vi "NML Power Monitoring Main.vi"(0 "Initialize":bool, 1 "Start":bool, 2 "Data Directory":path=path "C:/Test/NML_PM_Monitoring/Data", 3 "UUT Serial Number(s)":string="12345", 5 "UUT COUNT":i32(ring) items=["1", "2", "3", "4", "5", "6"], 7 "HRS":dbl, 9 "MINS":dbl=5.0, 11 "INTERVAL":dbl=30.0 caption="PROFILER (SEC)", 12 "Stop":bool, 13 "PM 2936R Settings":T3={"Wavelength nm"=633, "Range Select"=1, "Mode"=0, "Unit Select"=2, "Auto Select"=1, "Analog Filter"=4, "Digital Filter\n(int. 0 to 10000)"=0, "Filter"=1} {"Filter" items=["No filtering", "Analog filter", "Digital filter", "Analog and Digital filter"]; "Digital Filter\n(int. 0 to 10000)" min=0 max=10000; "Analog Filter" items=["None", "250 kHz", "12.5 kHz", "1 kHz", "5 kHz"]; "Auto Select" items=["Manual Range", "Auto Range"]; "Unit Select" items=["Amps", "Volts", "Watts", "Watts/cm2", "Joules", "Joules/cm2", "dBm"]; "Mode" items=["CW Cont.", "DC Single", "Integrate", "Peak-to-Peak Cont.", "Peak-to-Peak Single", "Pulse Continuous", "Pulse Single", "RMS"]; "Range Select" items=["Range 0", "Range 1", "Range 2", "Range 3", "Range 4", "Range 5", "Range 6", "Range 7"]; "Wavelength nm" min=0}) -> (4 "Status Message":string, 6 "XY Plot - 1 Trace":cluster{"Seconds":dbl[], "Data Array":dbl[]}[](graph), 8 "# of Samples":i32=10, 10 "Acquired Samples":i32, 14 "Data":dbl[][](array[numeric]), 15 "Error Out":errorcluster)   [LabVIEW 2017]
uses:
  Commands.ctl
  C:/Program Files (x86)/Newport/Newport USB Driver/Bin/UsbDllWrap.dll
  Program Files (x86)/Newport/Newport USB Driver/Bin/UsbDllWrap.dll
  Newport PowerMeter 2936R/Device State Control.ctl
panel:
  out "Time Array":string[](array[string])
  out "Date Array":string[](array[string])
  out "Collecting\n    Data":bool
  out "Start Time":timestamp
  out "PM Ready":bool
  out "PM Count":i32
  out "MINS Left":dbl format="%_3g"
  out "HRS Left":dbl
  out "Data Graphs":T1(tab)
  out "XY Plot - 2 Traces":cluster{"Seconds":dbl[], "Data Array":dbl[]}[](graph)
  out "XY Plot - 3 Traces":cluster{"Seconds":dbl[], "Data Array":dbl[]}[](graph)
  out "XY Plot - 4 Traces":cluster{"Seconds":dbl[], "Data Array":dbl[]}[](graph)
  out "XY Plot - 5 Traces":cluster{"Seconds":dbl[], "Data Array":dbl[]}[](graph)
  out "XY Plot - 6 Traces":cluster{"Seconds":dbl[], "Data Array":dbl[]}[](graph)
  out "Sample":dbl[](array[numeric])
  in  "Error In":errorcluster
  out "PM Ref":refnum<k24>[](array[refnum])
  in  "Commands":T2
  # "RUN  TIME"
  # "INTERVALS"
  # "PROFILER (SEC)"
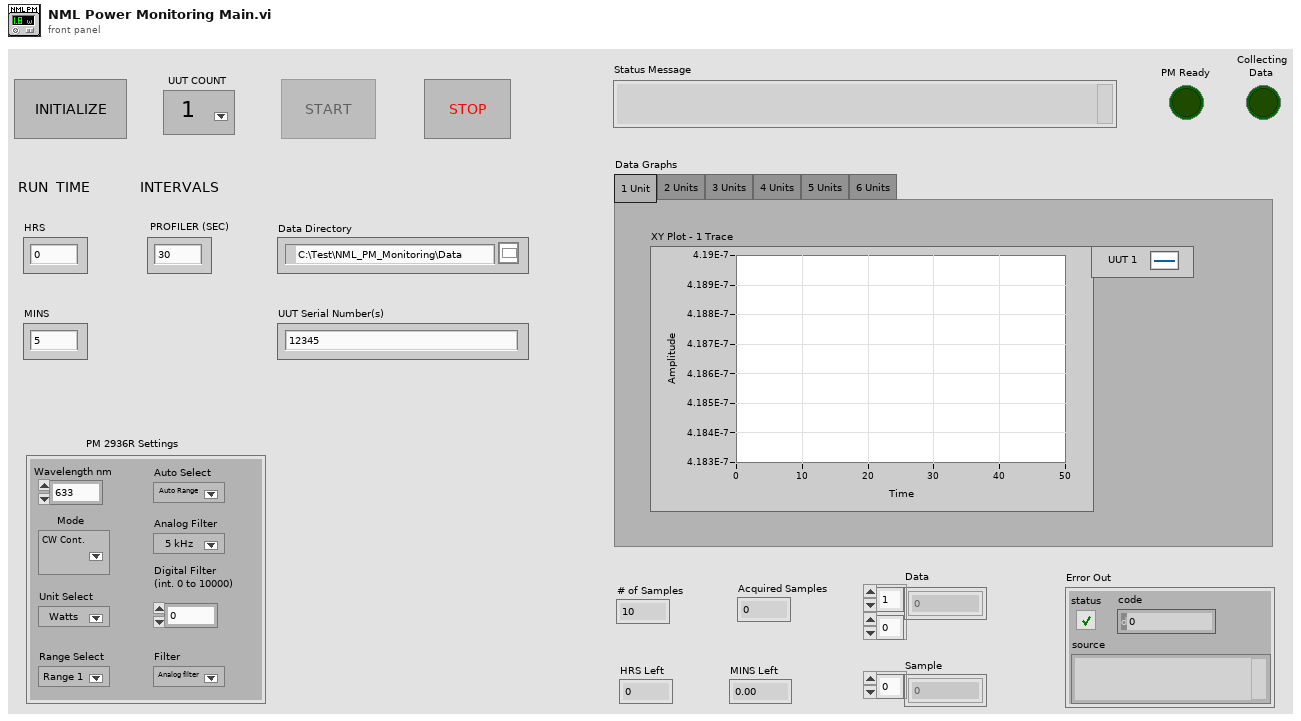
[diagram p1: front panel]
types:
  T1 = enum32{"1 Unit", "2 Units", "3 Units", "4 Units", "5 Units", "6 Units"}
  T2 = typedef "Commands.ctl" = enum16{"Idle", "Initialize", "Start", "Acquire Data", "Graph Data", "Store Data", "Halt"}
  T3 = cluster{"Wavelength nm":i32, "Range Select":i32, "Mode":i32, "Unit Select":i32, "Auto Select":i32, "Analog Filter":i32, "Digital Filter\n(int. 0 to 10000)":i32, "Filter":i32}
  T4 = enum8{"Enabled", "Disabled", "Disabled and Grayed Out"}
  T5 = typedef "Device State Control.ctl" = enum16{"Open", "Close", "Clear", "Set", "Reset", "Read", "Write", "Call"}
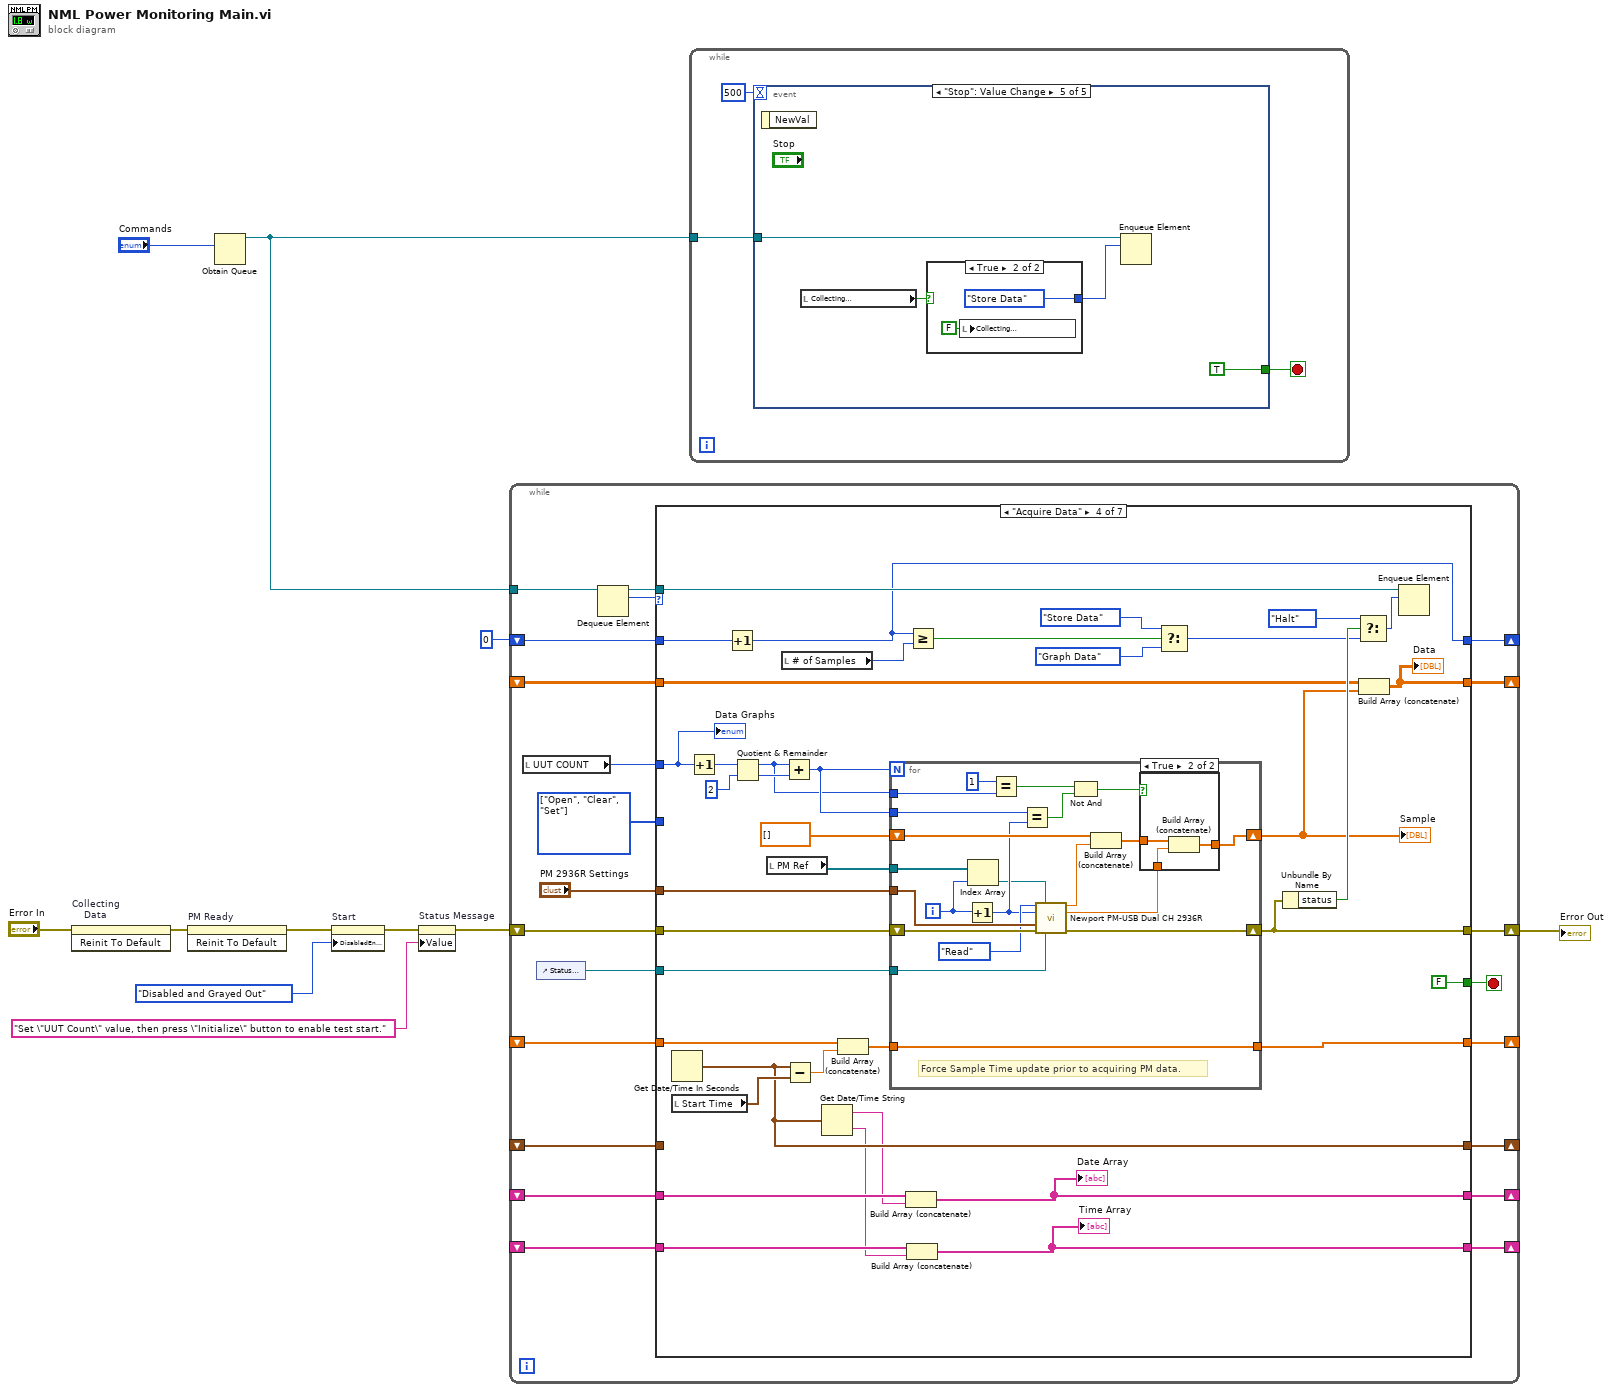
[diagram p0: block diagram]
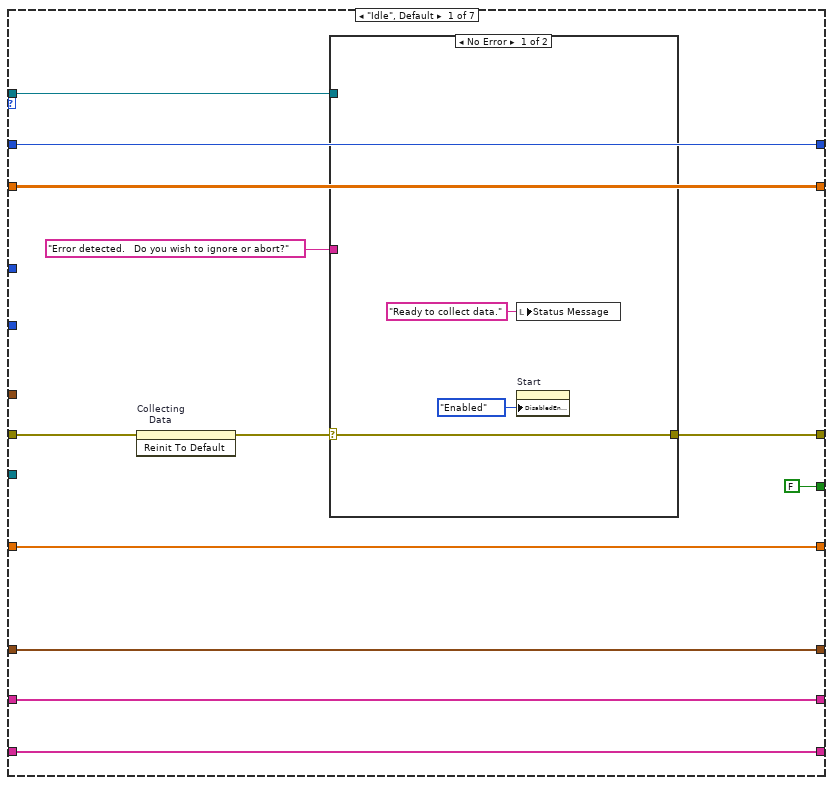
[diagram p2: hidden frame]
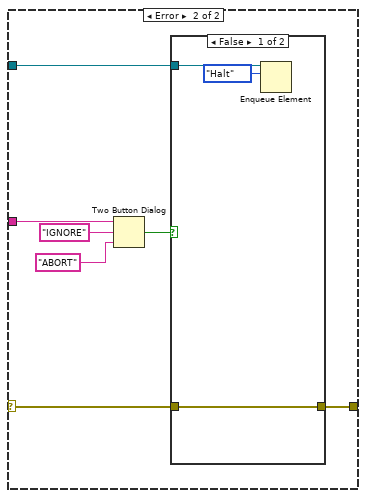
[diagram p3: hidden frame]
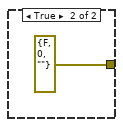
[diagram p4: hidden frame]
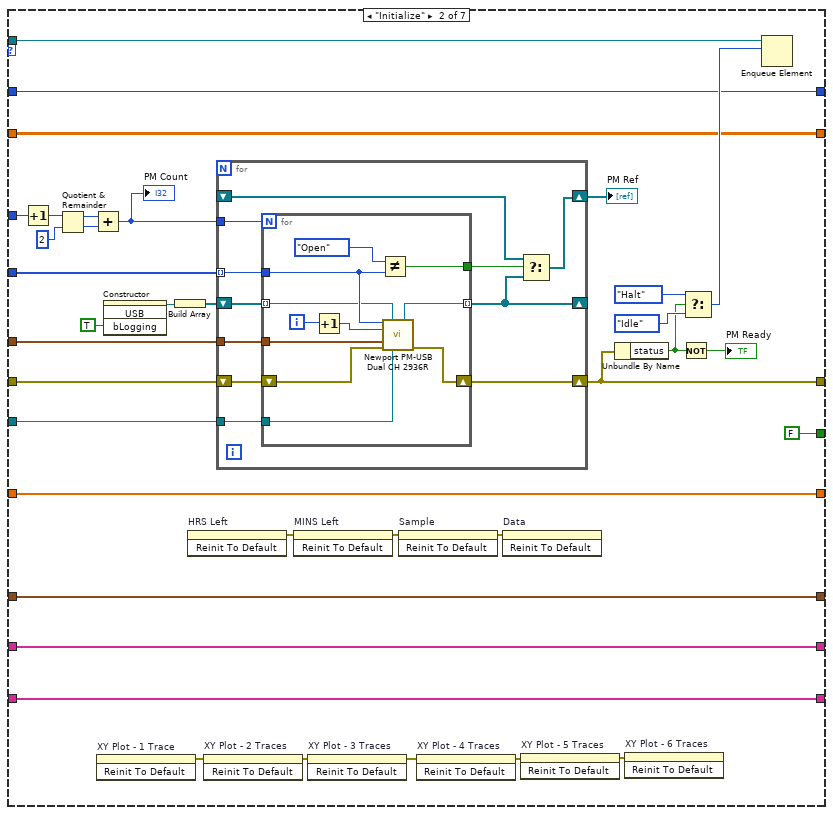
[diagram p5: hidden frame]
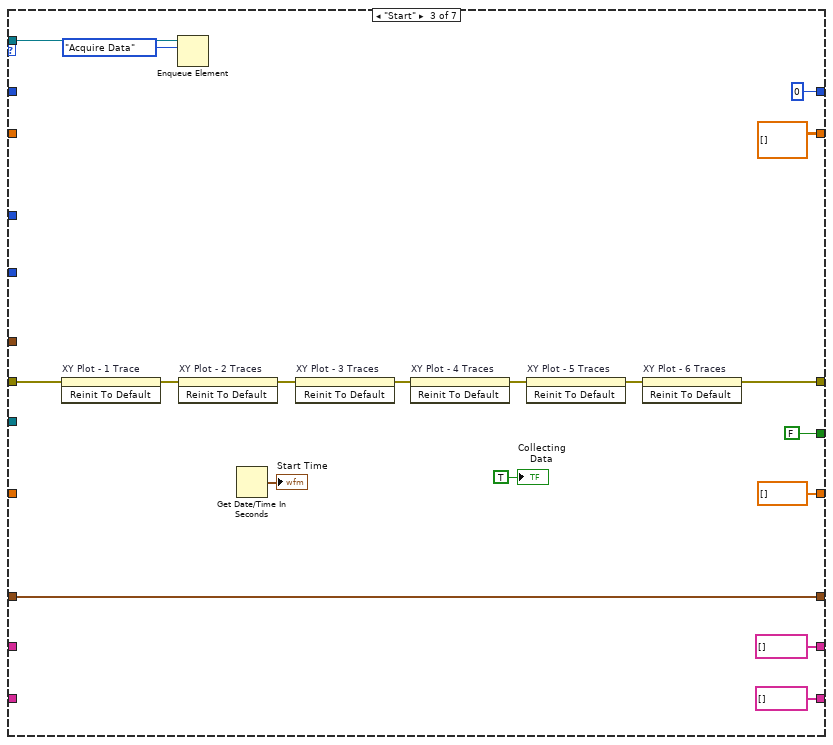
[diagram p6: hidden frame]
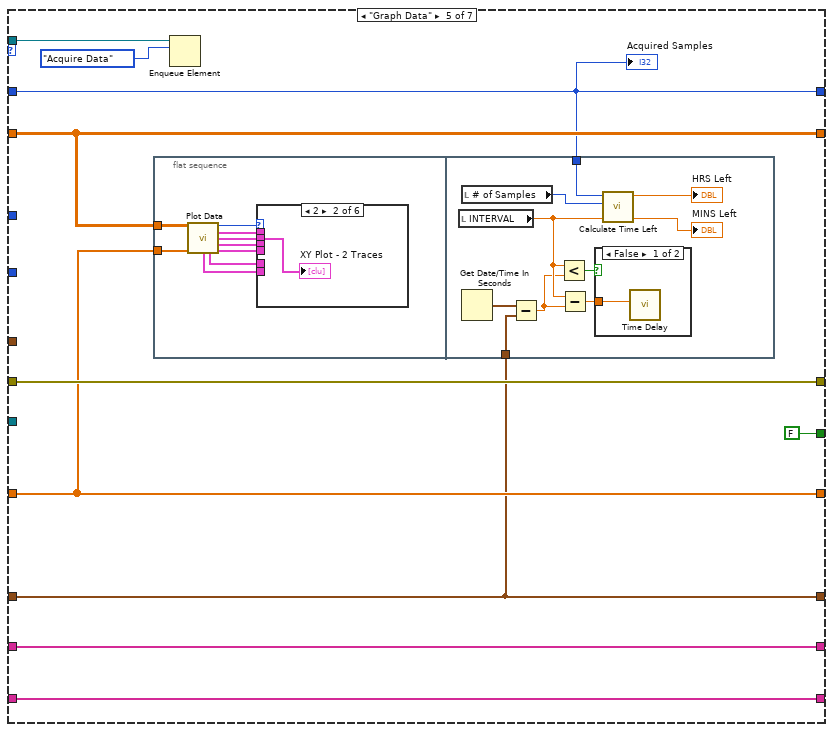
[diagram p8: hidden frame]
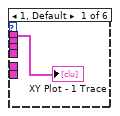
[diagram p9: hidden frame]
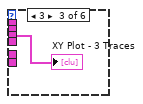
[diagram p10: hidden frame]
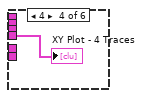
[diagram p11: hidden frame]
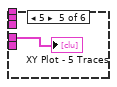
[diagram p12: hidden frame]
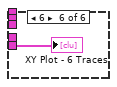
[diagram p13: hidden frame]
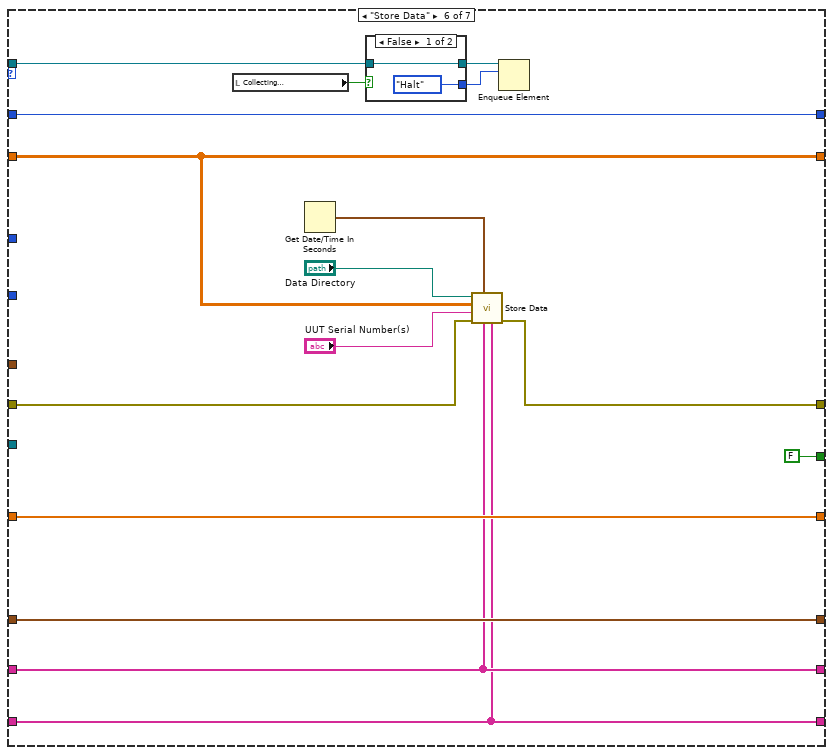
[diagram p15: hidden frame]
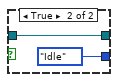
[diagram p16: hidden frame]
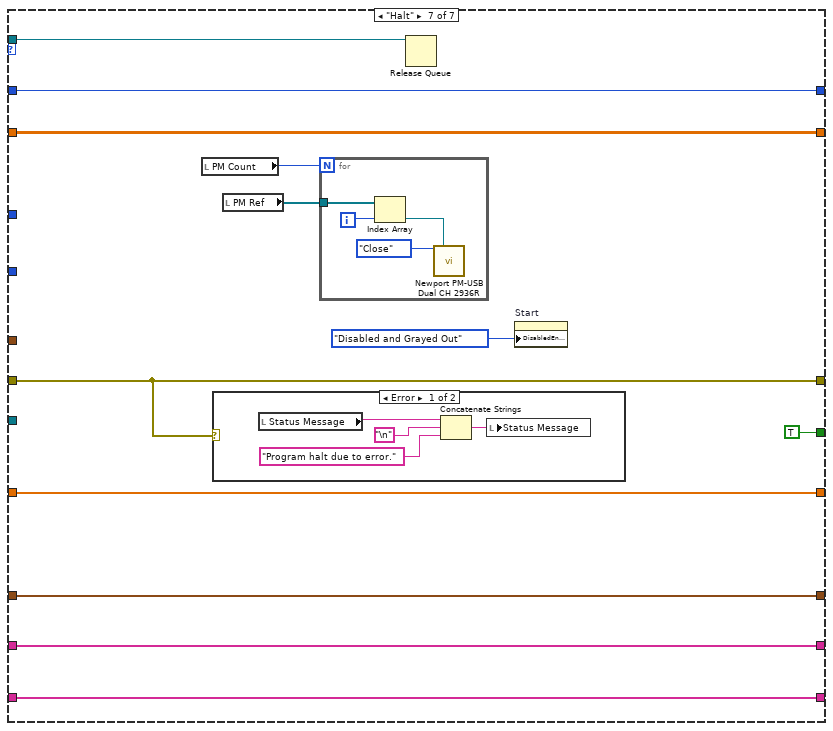
[diagram p17: hidden frame]
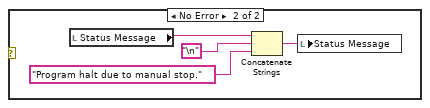
[diagram p18: hidden frame]
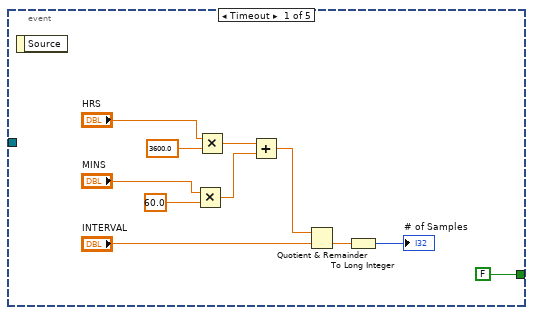
[diagram p19: hidden frame]
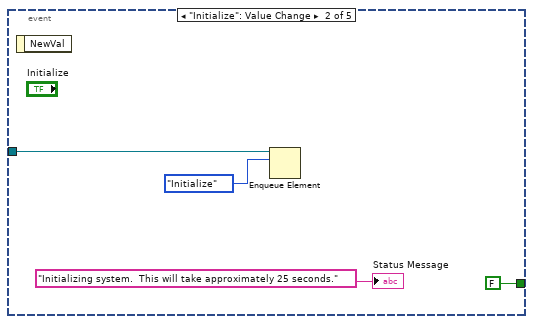
[diagram p20: hidden frame]
diagram:
  n1 = invoke on="Collecting\n    Data" class="Bool (strict)" method="Reinit To Default"(error in="Error In") -> (error out=w2:errorcluster)  [unwired: 2 in, 2 out]
  n2 = invoke on="PM Ready" class="Bool (strict)" method="Reinit To Default"(error in=w2) -> (error out=w5:errorcluster)  [unwired: 2 in, 2 out]
  n3 = Obtain Queue(element data type="Commands") -> (queue out=w10:refnum<queue>)  [unwired: 4 in, 2 out]
  n4 = property on="Start" class="Bool"(error in=w5, "DisabledEnum"=T4."Disabled and Grayed Out" ("Disabled")) -> (error out=w4:errorcluster)  [unwired: 1 in, 1 out]
  n5 = property on="Status Message" class="Str"(error in=w4, "Value"="Set \"UUT Count\" value, then press \"Initialize\" button to enable test start." ("Status Message")) -> (error out=w3:errorcluster)  [unwired: 1 in, 1 out]
  n6 = while {
    tunnel: w10 -> [w33]
    shift-right: [w28] -> w9
    shift-left: w3 -> [w29]
    shift-right: [w23] -> _
    shift-left: _ -> [w25]
    shift-right: [w22] -> _
    shift-left: 0 -> [w24]
    shift-right: [w20] -> _
    shift-left: _ -> [w21]
    shift-right: [w17] -> _
    shift-left: _ -> [w16]
    shift-right: [w15] -> _
    shift-left: _ -> [w14]
    shift-right: [w12] -> _
    shift-left: _ -> [w13]
    stop <- w19 stop-if-true
    w26 = T5[] [enum."Open", enum."Clear", enum."Set"] items=["Open", "Close", "Clear", "Set", "Reset", "Read", "Write", "Call"]
    n7 = local read "UUT COUNT"() -> (w18:i32)
    n8 = control-ref of="Status Message"() -> (w30:refnum<vi>)
    n9 = Dequeue Element(queue=w33) -> (queue out=w27:refnum<queue>, element=w32:T2)  [unwired: 2 in, 2 out]
    n10 = case shown="\"Acquire Data\"" w32 {
      tunnel: "PM 2936R Settings" -> [_ w95 _ w174 _ _ _]
      tunnel: w18 -> [_ w75 _ w145 _ _ _]
      tunnel: w30 -> [_ w94 _ w173 _ _ _]
      tunnel: w29 -> [w39 w93 w126 w172 w209 w237 w262]
      tunnel: [w45 w85 w125 w168 w209 w236 w262] -> w28
      tunnel: w27 -> [w34 w92 w133 w171 w205 w241 w264]
      tunnel: w26 -> [_ w91 _ _ _ _ _]
      tunnel: w25 -> [w43 w74 _ w160 w208 w244 w266]
      tunnel: w24 -> [w44 w81 _ w158 w206 w251 w267]
      tunnel: [w43 w74 dbl[][] [] w159 w208 w244 w266] -> w23
      tunnel: [w44 w81 0 w152 w206 w251 w267] -> w22
      tunnel: w21 -> [w42 w73 _ w151 w207 w243 w265]
      tunnel: [w42 w73 dbl[] [] w149 w207 w243 w265] -> w20
      tunnel: [FALSE FALSE FALSE FALSE FALSE FALSE TRUE] -> w19
      tunnel: [w40 w62 w121 w142 w202 w245 w258] -> w17
      tunnel: w16 -> [w40 w62 w121 _ w202 w245 w258]
      tunnel: [w37 w61 string[] [] w141 w201 w239 w257] -> w15
      tunnel: w14 -> [w37 w61 _ w140 w201 w239 w257]
      tunnel: w13 -> [w36 w60 _ w138 w200 w238 w256]
      tunnel: [w36 w60 string[] [] w137 w200 w238 w256] -> w12
      frame "Idle", Default {
        n11 = invoke on="Collecting\n    Data" class="Bool (strict)" method="Reinit To Default"(error in=w39) -> (error out=w38:errorcluster)  [unwired: 2 in, 2 out]
        n12 = case shown="No Error" w38 {
          selector: w38 -> [w47 w50]
          tunnel: [w47 w49] -> w45
          tunnel: "Error detected.   Do you wish to ignore or abort?" ("message") -> [_ w55]
          tunnel: w34 -> [_ w52]
          frame No Error {
            n13 = local write "Status Message"("Ready to collect data." ("Status Message")) -> ()
            n14 = property on="Start" class="Bool"("DisabledEnum"=T4."Enabled" ("Disabled")) -> ()  [unwired: 2 in, 2 out]
          }
          frame Error {
            n15 = Two Button Dialog(message=w55, 1:"ABORT" ("F button name (\"Cancel\")"), 2:"IGNORE" ("T button name (\"OK\")")) -> (T button?=w51:bool)
            n16 = case shown="False" w51 {
              tunnel: w52 -> [w58 _]
              tunnel: w50 -> [w56 _]
              tunnel: [w56 errorcluster {"status"=FALSE, "code"=0, "source"=""} ("error IO")] -> w49
              frame False {
                n17 = Enqueue Element(queue=w58, element=Commands."Halt") -> ()  [unwired: 2 in, 3 out]
              }
              frame True {
              }
            }
          }
        }
      }
      frame "Initialize" {
        n18 = Increment(x=w75) -> (x+1=w76:i32)
        n19 = Quotient & Remainder(x=w76, y=2) -> (x-y*floor(x/y)=w88:i32, floor(x/y)=w87:i32)
        n20 = Add(x=w88, y=w87) -> (x+y=w86:i32)
        "PM Count" <- w86
        n21 = invoke on="XY Plot - 1 Trace" class="XYGraph (strict)" method="Reinit To Default"() -> (error out=w66:errorcluster)  [unwired: 3 in, 2 out]
        n22 = constructor class="USB"("bLogging"=TRUE) -> (reference out=w79:refnum<k24>)  [unwired: 3 in, 3 out]
        n23 = Build Array(w79) -> (w77:refnum<k24>[])
        n24 = invoke on="HRS Left" class="DigNum (strict)" method="Reinit To Default"() -> (error out=w70:errorcluster)  [unwired: 3 in, 2 out]
        n25 = invoke on="XY Plot - 2 Traces" class="XYGraph (strict)" method="Reinit To Default"(error in=w66) -> (error out=w67:errorcluster)  [unwired: 2 in, 2 out]
        n26 = for {
          tunnel: w95 -> [w106]
          tunnel: w86 -> [w105]
          tunnel: w94 -> [w104]
          shift-right: [w98] -> w85
          shift-left: w93 -> [w99]
          tunnel: w91 -> [w103] mode=indexing
          shift-right: [w100] -> w90
          shift-left: _ -> [w101]
          shift-right: [w97] -> _
          shift-left: w77 -> [w96]
          n27 = for {
            N: w105 -> [_]
            tunnel: w106 -> [w117]
            tunnel: [w114] -> w97 mode=indexing
            tunnel: w104 -> [w113]
            tunnel: w103 -> [w112]
            tunnel: [w110] -> w102
            shift-right: [w108] -> w98
            shift-left: w99 -> [w109]
            tunnel: w96 -> [w107] mode=indexing
            i -> [w116]
            n28 = Increment(x=w116) -> (x+1=w115:i32)
            n29 = Not Equal?(x=Device_State_Control."Open" ("Device State Control"), y=w112) -> (x != y?=w110:bool)
            n30 = call "Newport PM-USB Dual CH 2936R.vi"("Device State Control"=w112, "2936R Ref In"=w107, "USB Address"=w115, "PowerMeter 2936R Settings"=w117, "2936R error in"=w109, "Msg Ctl Refnum"=w113) -> ("2936R Ref Out"=w114:refnum<k24>, "2936R error out"=w108:errorcluster)  [unwired: 2 in, 6 out]
          }
          n31 = Select(t=w101, s=w102, f=w97) -> (s? t:f=w100:refnum<k24>[])
        }
        "PM Ref" <- w90
        n32 = invoke on="MINS Left" class="DigNum (strict)" method="Reinit To Default"(error in=w70) -> (error out=w69:errorcluster)  [unwired: 2 in, 2 out]
        n33 = invoke on="XY Plot - 3 Traces" class="XYGraph (strict)" method="Reinit To Default"(error in=w67) -> (error out=w63:errorcluster)  [unwired: 2 in, 2 out]
        n34 = invoke on="Sample" class="Arr (strict)" method="Reinit To Default"(error in=w69) -> (error out=w68:errorcluster)  [unwired: 2 in, 2 out]
        n35 = invoke on="XY Plot - 4 Traces" class="XYGraph (strict)" method="Reinit To Default"(error in=w63) -> (error out=w64:errorcluster)  [unwired: 2 in, 2 out]
        n36 = invoke on="Data" class="Arr (strict)" method="Reinit To Default"(error in=w68) -> ()  [unwired: 2 in, 3 out]
        n37 = invoke on="XY Plot - 5 Traces" class="XYGraph (strict)" method="Reinit To Default"(error in=w64) -> (error out=w65:errorcluster)  [unwired: 2 in, 2 out]
        n38 = Unbundle By Name(w85) -> ("status"=w72:bool)
        n39 = invoke on="XY Plot - 6 Traces" class="XYGraph (strict)" method="Reinit To Default"(error in=w65) -> ()  [unwired: 2 in, 3 out]
        n40 = Not(x=w72) -> (.not. x?=→"PM Ready":bool)
        n41 = Select(t=Commands."Halt" ("element"), s=w72, f=Commands."Idle" ("element")) -> (s? t:f=w82:T2)
        n42 = Enqueue Element(queue=w92, element=w82) -> ()  [unwired: 2 in, 3 out]
      }
      frame "Start" {
        n43 = invoke on="XY Plot - 1 Trace" class="XYGraph (strict)" method="Reinit To Default"(error in=w126) -> (error out=w131:errorcluster)  [unwired: 2 in, 2 out]
        n44 = Enqueue Element(queue=w133, element=Commands."Acquire Data") -> ()  [unwired: 2 in, 3 out]
        n45 = invoke on="XY Plot - 2 Traces" class="XYGraph (strict)" method="Reinit To Default"(error in=w131) -> (error out=w130:errorcluster)  [unwired: 2 in, 2 out]
        n46 = Get Date/Time In Seconds() -> (seconds since 1Jan1904=→"Start Time":timestamp)
        n47 = invoke on="XY Plot - 3 Traces" class="XYGraph (strict)" method="Reinit To Default"(error in=w130) -> (error out=w129:errorcluster)  [unwired: 2 in, 2 out]
        n48 = invoke on="XY Plot - 4 Traces" class="XYGraph (strict)" method="Reinit To Default"(error in=w129) -> (error out=w128:errorcluster)  [unwired: 2 in, 2 out]
        n49 = invoke on="XY Plot - 5 Traces" class="XYGraph (strict)" method="Reinit To Default"(error in=w128) -> (error out=w127:errorcluster)  [unwired: 2 in, 2 out]
        n50 = invoke on="XY Plot - 6 Traces" class="XYGraph (strict)" method="Reinit To Default"(error in=w127) -> (error out=w125:errorcluster)  [unwired: 2 in, 2 out]
        "Collecting\n    Data" <- TRUE ("Collecting Data")
      }
      frame "Acquire Data" {
        n51 = Get Date/Time In Seconds() -> (seconds since 1Jan1904=w142:timestamp)
        n52 = local read "Start Time"() -> (w144:timestamp)
        n53 = Increment(x=w145) -> (x+1=w146:i32)
        n54 = Increment(x=w158) -> (x+1=w152:i32)
        n55 = Quotient & Remainder(x=w146, y=2) -> (x-y*floor(x/y)=w162:i32, floor(x/y)=w169:i32)
        n56 = local read "PM Ref"() -> (w147:refnum<k24>[])
        n57 = local read "# of Samples"() -> (w157:i32)
        n58 = Add(x=w162, y=w169) -> (x+y=w163:i32)
        n59 = Subtract(x=w142, y=w144) -> (x-y=w143:dbl)
        n60 = Get Date/Time String(seconds (now)=w142) -> (date string=w139:string, time string=w136:string)  [unwired: 2 in]
        n61 = Build Array (concatenate)(w151, w143) -> (w150:dbl[])
        n62 = for {
          N: w163 -> [_]
          tunnel: w174 -> [w195]
          tunnel: w173 -> [w194]
          shift-right: [w192] -> w168
          shift-left: w172 -> [w193]
          shift-right: [w179] -> w161
          shift-left: dbl[] [] -> [w190]
          tunnel: w163 -> [w188]
          tunnel: w162 -> [w186]
          tunnel: w150 -> [w178]
          tunnel: [w178] -> w149
          tunnel: w147 -> [w176]
          i -> [w177]
          # "Force Sample Time update prior to acquiring PM data."
          n63 = Increment(x=w177) -> (x+1=w187:i32)
          n64 = Index Array(array=w176, index=w177) -> (element=w175:refnum<k24>)
          n65 = Equal?(x=1, y=w186) -> (x = y?=w184:bool)
          n66 = Equal?(x=w188, y=w187) -> (x = y?=w183:bool)
          n67 = call "Newport PM-USB Dual CH 2936R.vi"("Device State Control"=Device_State_Control."Read", "2936R Ref In"=w175, "USB Address"=w187, "PowerMeter 2936R Settings"=w195, "2936R error in"=w193, "Msg Ctl Refnum"=w194) -> ("CH1, W"=w189:dbl, "Ch2, W"=w180:dbl, "2936R error out"=w192:errorcluster)  [unwired: 2 in, 5 out]
          n68 = Not And(1:w183, 2:w184) -> (0:w182:bool)
          n69 = Build Array (concatenate)(w190, w189) -> (w181:dbl[])
          n70 = case shown="True" w182 {
            tunnel: w181 -> [w196 w199]
            tunnel: w180 -> [_ w198]
            tunnel: [w196 w197] -> w179
            frame False {
            }
            frame True {
              n71 = Build Array (concatenate)(w199, w198) -> (w197:dbl[])
            }
          }
        }
        "Sample" <- w161
        n72 = Build Array (concatenate)(w140, w139) -> (w141:string[])
        "Date Array" <- w141
        n73 = Build Array (concatenate)(w138, w136) -> (w137:string[])
        "Time Array" <- w137
        n74 = Greater Or Equal?(x=w152, y=w157) -> (x >= y?=w155:bool)
        n75 = Select(t=Commands."Store Data" ("element"), s=w155, f=Commands."Graph Data" ("element")) -> (s? t:f=w153:T2)
        n76 = Unbundle By Name(w168) -> ("status"=w166:bool)
        n77 = Select(t=Commands."Halt" ("element"), s=w166, f=w153) -> (s? t:f=w165:T2)
        n78 = Build Array (concatenate)(w160, w161) -> (w159:dbl[][])
        "Data" <- w159
        n79 = Enqueue Element(queue=w171, element=w165) -> ()  [unwired: 2 in, 3 out]
        "Data Graphs" <- w145
      }
      frame "Graph Data" {
        n80 = flat-sequence {
          tunnel: w208 -> [w218]
          tunnel: w207 -> [w217]
          tunnel: w206 -> [w231]
          tunnel: w202 -> [w225]
          frame #0 {
            n81 = call "Plot Data.vi"("Data Array"=w218, "Seconds"=w217) -> ("Number of Plots"=w216:i32, "XY Plot - 1 Trace"=w215:cluster{"Seconds":dbl[], "Data Array":dbl[]}[], "XY Plot - 2 Traces"=w214:cluster{"Seconds":dbl[], "Data Array":dbl[]}[], "XY Plot - 3 Traces"=w213:cluster{"Seconds":dbl[], "Data Array":dbl[]}[], "XY Plot - 6 Traces"=w210:cluster{"Seconds":dbl[], "Data Array":dbl[]}[], "XY Plot - 5 Traces"=w211:cluster{"Seconds":dbl[], "Data Array":dbl[]}[], "XY Plot - 4 Traces"=w212:cluster{"Seconds":dbl[], "Data Array":dbl[]}[])  [unwired: 7 in]
            n82 = case shown="2" w216 {
              tunnel: w215 -> [w219 _ _ _ _ _]
              tunnel: w214 -> [_ w220 _ _ _ _]
              tunnel: w213 -> [_ _ w221 _ _ _]
              tunnel: w212 -> [_ _ _ w222 _ _]
              tunnel: w211 -> [_ _ _ _ w223 _]
              tunnel: w210 -> [_ _ _ _ _ w224]
              frame 1, Default {
                "XY Plot - 1 Trace" <- w219
              }
              frame 2 {
                "XY Plot - 2 Traces" <- w220
              }
              frame 3 {
                "XY Plot - 3 Traces" <- w221
              }
              frame 4 {
                "XY Plot - 4 Traces" <- w222
              }
              frame 5 {
                "XY Plot - 5 Traces" <- w223
              }
              frame 6 {
                "XY Plot - 6 Traces" <- w224
              }
            }
          }
          frame #1 {
            n83 = local read "INTERVAL"() -> (w229:dbl)
            n84 = local read "# of Samples"() -> (w232:i32)
            n85 = Get Date/Time In Seconds() -> (seconds since 1Jan1904=w234:timestamp)
            n86 = Subtract(x=w234, y=w225) -> (x-y=w228:dbl)
            n87 = Less?(x=w229, y=w228) -> (x < y?=w233:bool)
            n88 = Subtract(x=w229, y=w228) -> (x-y=w230:dbl)
            n89 = case shown="False" w233 {
              tunnel: w230 -> [w235 _]
              frame False {
                n90 = call "Time Delay"("Delay Time (s)"=w235) -> ()  [unwired: 10 in, 1 out]
              }
              frame True {
              }
            }
            n91 = call "Calculate Time Left.vi"("Interval"=w229, "Total Samples"=w232, "Acquired Samples"=w231) -> ("MINS Left"=→"MINS Left":dbl, "HRS Left"=→"HRS Left":dbl)  [unwired: 7 in]
          }
        }
        n92 = Enqueue Element(queue=w205, element=Commands."Acquire Data") -> ()  [unwired: 2 in, 3 out]
        "Acquired Samples" <- w206
      }
      frame "Store Data" {
        n93 = local read "Collecting\n    Data"() -> (w242:bool)
        n94 = Get Date/Time In Seconds() -> (seconds since 1Jan1904=w248:timestamp)
        n95 = case shown="False" w242 {
          tunnel: [Commands."Halt" ("element") Commands."Idle" ("element")] -> w247
          tunnel: w241 -> [w253 w254]
          tunnel: [w253 w254] -> w240
          frame False {
          }
          frame True {
          }
        }
        n96 = call "Store Data.vi"("Time Array"=w238, "Date Array"=w239, "Time Stamp"=w248, "Error In"=w237, "S/N"="UUT Serial Number(s)", "Data Array"=w244, "Data Dir"="Data Directory") -> ("Error Out"=w236:errorcluster)  [unwired: 3 in, 1 out]
        n97 = Enqueue Element(queue=w240, element=w247) -> ()  [unwired: 2 in, 3 out]
      }
      frame "Halt" {
        n98 = local read "PM Count"() -> (w260:i32)
        n99 = case shown="Error" w262 {
          frame Error {
            n100 = local read "Status Message"() -> (w275:string)
            n101 = Concatenate Strings(w275, "\n", "Program halt due to error." ("Status Message")) -> (w273:string)
            n102 = local write "Status Message"(w273) -> ()
          }
          frame No Error {
            n103 = local read "Status Message"() -> (w279:string)
            n104 = Concatenate Strings(w279, "\n", "Program halt due to manual stop." ("Status Message")) -> (w277:string)
            n105 = local write "Status Message"(w277) -> ()
          }
        }
        n106 = local read "PM Ref"() -> (w261:refnum<k24>[])
        n107 = for {
          N: w260 -> [_]
          tunnel: w261 -> [w270]
          i -> [w269]
          n108 = Index Array(array=w270, index=w269) -> (element=w268:refnum<k24>)
          n109 = call "Newport PM-USB Dual CH 2936R.vi"("Device State Control"=Device_State_Control."Close", "2936R Ref In"=w268) -> ()  [unwired: 6 in, 8 out]
        }
        n110 = Release Queue(queue=w264) -> ()  [unwired: 2 in, 3 out]
        n111 = property on="Start" class="Bool"("DisabledEnum"=T4."Disabled and Grayed Out" ("Disabled")) -> ()  [unwired: 2 in, 2 out]
      }
    }
  }
  "Error Out" <- w9
  n112 = while {
    tunnel: w10 -> [w282]
    stop <- w281 stop-if-true
    n113 = event shown="[4] \"Stop\": Value Change" {
      selector: _ -> [_ _ _ _ _]
      dyn-events: _ -> [_ _ _ _ _]
      timeout: 500 -> [_ _ _ _ _]
      tunnel: w282 -> [_ w297 w298 w310 w314]
      tunnel: [FALSE FALSE FALSE FALSE TRUE] -> w281
      event Timeout {
        n114 = event-data() -> ()  [unwired: 1 in, 1 out]
        n115 = Multiply(x="MINS", y=60.0) -> (x*y=w292:dbl)
        n116 = Multiply(x="HRS", y=3600.0) -> (x*y=w293:dbl)
        n117 = Add(x=w293, y=w292) -> (x+y=w291:dbl)
        n118 = Quotient & Remainder(x=w291, y="INTERVAL") -> (floor(x/y)=w290:dbl)  [unwired: 1 out]
        n119 = To Long Integer(number=w290) -> (32bit integer=→"# of Samples":i32)
      }
      event "Initialize": Value Change {
        n120 = event-data() -> ()  [unwired: 1 in, 1 out]
        n121 = Enqueue Element(queue=w297, element=Commands."Initialize") -> ()  [unwired: 2 in, 3 out]
        "Status Message" <- "Initializing system.  This will take approximately 25 seconds." ("Status Message")
      }
      event "UUT COUNT": Value Change {
        n122 = event-data() -> ()  [unwired: 1 in, 1 out]
        n123 = local read "PM Ready"() -> (w299:bool)
        n124 = case shown="True" w299 {
          tunnel: "Program must be restarted to change UUT count." ("Status Message") -> [_ w304]
          tunnel: w298 -> [_ w303]
          frame False {
          }
          frame True {
            n125 = local read "Status Message"() -> (w306:string)
            n126 = Enqueue Element(queue=w303, element=Commands."Halt") -> ()  [unwired: 2 in, 3 out]
            n127 = Concatenate Strings(w306, "\n", w304) -> (w307:string)
            n128 = local write "Status Message"(w307) -> ()
          }
        }
      }
      event "Start": Value Change {
        n129 = event-data() -> ()  [unwired: 1 in, 1 out]
        n130 = local write "Status Message"("Collecting Data" ("Status Message")) -> ()
        n131 = Enqueue Element(queue=w310, element=Commands."Start") -> ()  [unwired: 2 in, 3 out]
      }
      event "Stop": Value Change {
        n132 = event-data() -> ()  [unwired: 1 in, 1 out]
        n133 = local read "Collecting\n    Data"() -> (w312:bool)
        n134 = case shown="True" w312 {
          tunnel: [Commands."Halt" ("element") Commands."Store Data" ("element")] -> w315
          frame False {
          }
          frame True {
            n135 = local write "Collecting\n    Data"(FALSE ("Collecting Data")) -> ()
          }
        }
        n136 = Enqueue Element(queue=w314, element=w315) -> ()  [unwired: 2 in, 3 out]
      }
    }
  }
